vi "Omega & Angular Velocity Calc.vi"(4 "omega and angular velocity calc input array":dbl[](array[numeric])) -> (1 "omega and angular velocity calc output array":dbl[](array[numeric]))   [LabVIEW 2015]
uses:
  <vilib>/addons/control/pid/pid.llb/PID (DBL).vi
  <vilib>/addons/control/pid/NI_PID_pid.lvlib
panel:
  in  "Avg R Dist Old":dbl
  out "Desired Velocity":dbl
  out "Omega":dbl format="%.2f"
  out "Phi desired":dbl
  in  "Desired X Velocity u1":dbl format="%#_13g"
  in  "Desired Y Velocity u2":dbl format="%#_13g"
  in  "Phi Current":dbl format="%#_13g"
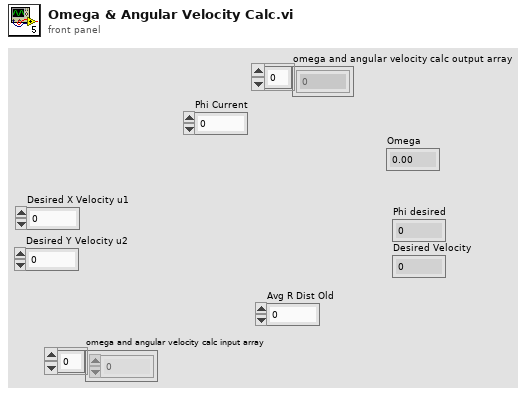
[diagram p1: front panel]
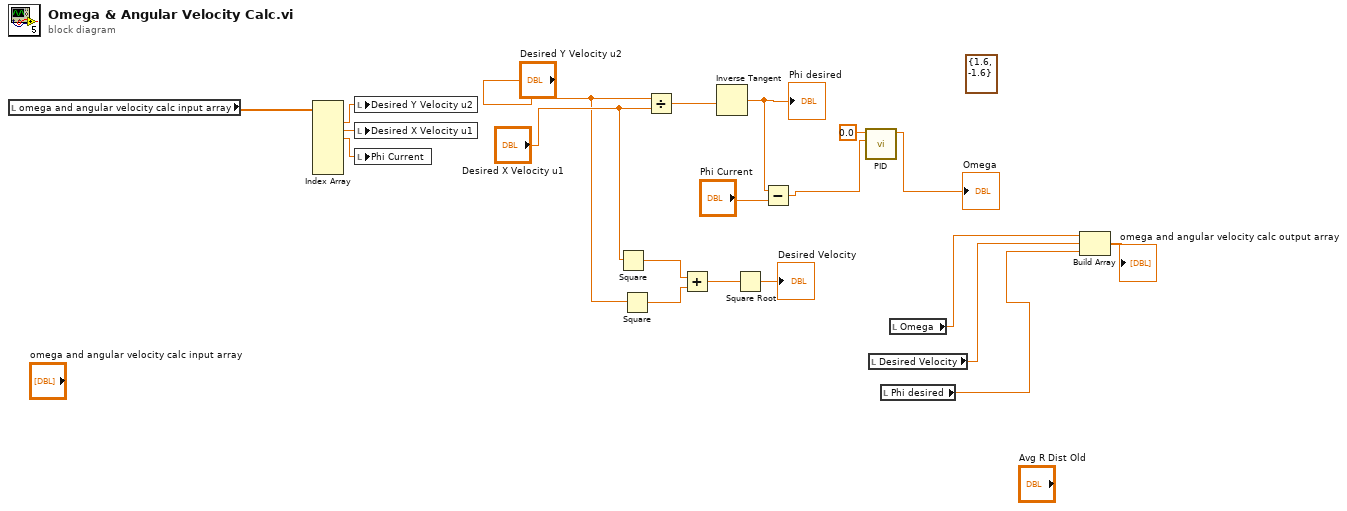
[diagram p0: block diagram]
diagram:
  (unwired) cluster{"output high":dbl, "output low":dbl} {"output high"=1.6, "output low"=-1.6} ("output range")
  n1 = local read "omega and angular velocity calc input array"() -> (w10:dbl[])
  n2 = Index Array(array=w10) -> (element #1=w9:dbl, element #2=w8:dbl, element #3=w7:dbl)  [unwired: 7 in, 4 out]
  n3 = local write "Desired Y Velocity u2"(w9) -> ()
  n4 = local write "Desired X Velocity u1"(w8) -> ()
  n5 = local write "Phi Current"(w7) -> ()
  n6 = Square(x="Desired X Velocity u1") -> (x^2=w18:dbl)
  n7 = Square(x="Desired Y Velocity u2") -> (x^2=w17:dbl)
  n8 = Divide(x="Desired Y Velocity u2", y="Desired X Velocity u1") -> (x/y=w20:dbl)
  n9 = Add(x=w18, y=w17) -> (x+y=w16:dbl)
  n10 = Inverse Tangent(1:w20) -> (0:w4:dbl)
  "Phi desired" <- w4
  n11 = Square Root(x=w16) -> (sqrt(x)=→"Desired Velocity":dbl)
  n12 = Subtract(x=w4, y="Phi Current") -> (x-y=w2:dbl)
  n13 = call-poly <vilib>:"PID.vi"("process variable"=w2, "setpoint"=0.0) -> ("output"=→"Omega":dbl)  [unwired: 8 in, 1 out]
  n14 = local read "Desired Velocity"() -> (w13:dbl)
  n15 = local read "Phi desired"() -> (w12:dbl)
  n16 = local read "Omega"() -> (w14:dbl)
  n17 = Build Array(w14, w13, w12) -> (→"omega and angular velocity calc output array":dbl[])
